vi "IDS_system_setInitMode.vi"(2 "error in (no error)":errorcluster, 3 "InitMode":i32, 4 "deviceHandle":i32) -> (0 "error out":errorcluster, 1 "deviceHandle out":i32)   [LabVIEW 2016]
doc: "int IDS_DLL IDS_rt_setRtOutMode(const int32_t rtOutMode);"
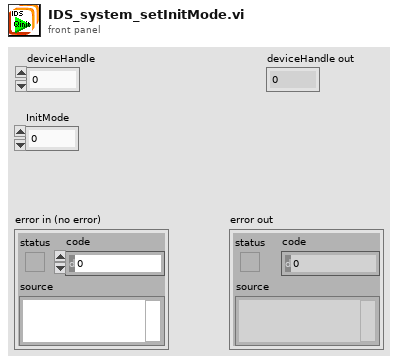
[diagram p1: front panel]
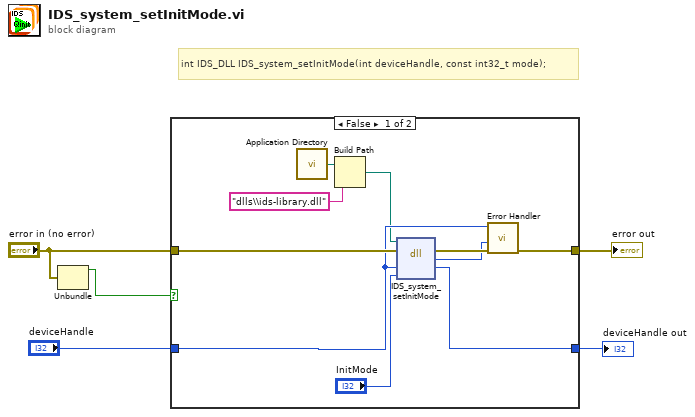
[diagram p0: block diagram]
diagram:
  # "int IDS_DLL IDS_system_setInitMode(int deviceHandle, const int32_t mode);"
  n1 = Unbundle("error in (no error)") -> ("status"=w1:bool)  [unwired: 2 out]
  n2 = case shown="False" w1 {
    tunnel: "error in (no error)" -> [w14 w17]
    tunnel: [w15 w17] -> w5
    tunnel: "deviceHandle" -> [w9 w16]
    tunnel: [w11 w16] -> w3
    frame False {
      n3 = call <vilib>:"Application Directory.vi"() -> ("Application Directory"=w8:path)
      n4 = Build Path(base path=w8, name or relative path="dlls\\ids-library.dll" ("ipAddress")) -> (appended path=w6:path)
      n5 = dll-call lib="C:/Users/matheus/Desktop/LabVIEW_Draft_V1.6.0/dlls/ids-library.*" fn="IDS_system_setInitMode"(path in=w6, error in=w14, "deviceHandle"=w9, "mode"="InitMode") -> (error out=w13:errorcluster, "return type"=w10:i32, "deviceHandle"=w11:i32)  [unwired: 2 in, 1 out]
      n6 = call "Error Handler.vi"("error in (no error)"=w13, "error code"=w10, "deviceHandle"=w9) -> ("error out"=w15:errorcluster)  [unwired: 7 in, 1 out]
    }
    frame True {
    }
  }
  "error out" <- w5
  "deviceHandle out" <- w3
